vi "solar_type Message to Script.vi"(6 "Array Delimiters (1D,2D)":string[](array[string]), 7 "Type (CMD)":enum8{"CMD", "TLM"}(ring), 8 "error in (no error)":errorcluster, 9 "Data":variant, 10 "Packet":string, 11 "Target (\"\")":string) -> (0 "error out":errorcluster, 3 "String":string)   [LabVIEW 2018]
doc: "This converts a SOLAR variant message to script string. Formatted as:\n<b>CMD|TLM.TARGET:PACKET{\nTYPE:VALUE,\nTYPE:'VALUE',\nTYPE|ENUM0|ENUM1|...:VALUE,\nTYPE_1D:'1,2,3',\nTYPE_2D:'1,2,3;4,5,6'}</b>\n\n<b>TYPE</b>= I8, I16, I32, I64, U8, U16, U32, U64, U8_ENUM, U16_ENUM, U32_ENUM, SGL, DBL, BOOL, STR, PATH, TIME\nTYPE_1D: 1D array (comma ',' delimited) Ex: DBL_1D:'1.23,4.567,8.92'\nTYPE_2D: 2D array (comma ',' & semicolon ';' delimited) Ex: I32_2D:'1,2,3;4,5,6'\nTYPE_ENUM: Enum with type items (pipe '|' delimited) Ex: U16_ENUM|Item 1|Item 2|Item 3:'Item 2'\n\nMyTarget:MyCMD{\nI32:-1234,\nSTR:'Hello World',\nU16_ENUM|Item1|Item2|Item3:'Item2',\nBOOL:true,\nTIME:'yyyy-mm-dd_hh:mm:ss.uuuuuu',\nPATH:'C:\\Data\\test.txt',\nU8_2D:'1,2,3;4,5,6'}"
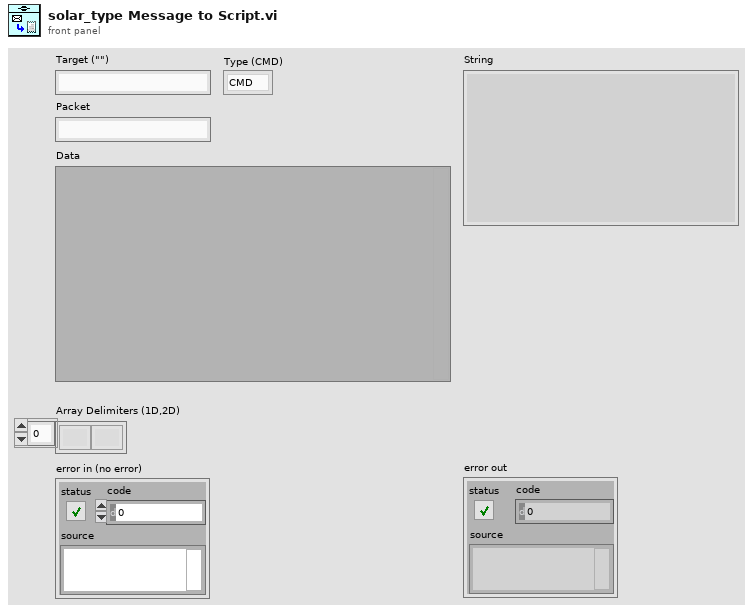
[diagram p1: front panel]
types:
  T1 = typedef "solar_type Item.ctl" = cluster{"Item":string, "Type":T2, "Value":variant, "States":string[]}
  T2 = typedef "solar_type Item Type.ctl" = enum16{"NULL", "UNKNOWN", "CLUSTER", "I8", "I16", "I32", "I64", "U8", "U16", "U32", "U64", "U8_ENUM", "U16_ENUM", "U32_ENUM", "SGL", "DBL", "BOOLEAN", "STRING", "PATH", "VISA", "TAG", "TIME", "I8_1D", "I16_1D", "I32_1D", "I64_1D", "U8_1D", "U16_1D", "U32_1D", "U64_1D", "U8_ENUM_1D", "U16_ENUM_1D", "U32_ENUM_1D", "SGL_1D", "DBL_1D", "BOOLEAN_1D", "STRING_1D", "PATH_1D", "VISA_1D", "TAG_1D", "TIME_1D", "I8_2D", "I16_2D", "I32_2D", "I64_2D", "U8_2D", "U16_2D", "U32_2D", "U64_2D", "U8_ENUM_2D", "U16_ENUM_2D", "U32_ENUM_2D", "SGL_2D", "DBL_2D", "BOOLEAN_2D", "STRING_2D", "PATH_2D", "VISA_2D", "TAG_2D", "TIME_2D"}
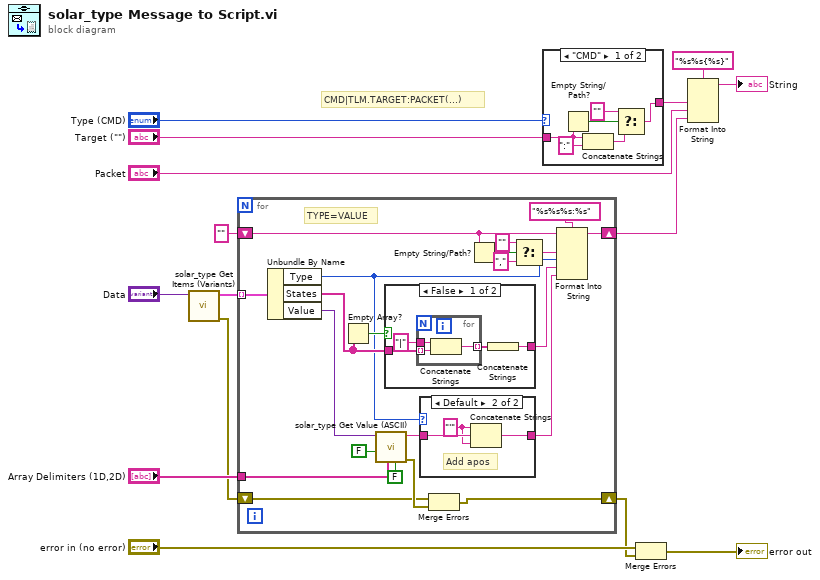
[diagram p0: block diagram]
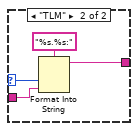
[diagram p2: hidden frame]
diagram:
  # "CMD|TLM.TARGET:PACKET(...)"
  n1 = call "solar_type Get Items (Variants).vi"("Variant"="Data") -> ("error out"=w2:errorcluster, "Items"=w6:T1[])  [unwired: 7 in, 2 out]
  n2 = for {
    tunnel: w6 -> [w36] mode=indexing
    tunnel: "Array Delimiters (1D,2D)" -> [w34]
    shift-right: [w29] -> w3
    shift-left: "" -> [w26]
    shift-right: [w17] -> w1
    shift-left: w2 -> [w16]
    # "TYPE=VALUE"
    n3 = Unbundle By Name(w36) -> ("Type"=w19:T2, "States"=w31:string[], "Value"=w33:variant)
    n4 = Empty Array?(array=w31) -> (empty?=w30:bool)
    n5 = call "solar_type Get Value (ASCII).vi"("Boolean as 0,1? (F)"=FALSE, "ArrayDelimiters (1D,2D)"=w34, "Use Enum Names? (F)"=FALSE, "Variant"=w33) -> ("error out"=w18:errorcluster, "Value (ASCII)"=w22:string)  [unwired: 5 in, 1 out]
    n6 = case shown="False" w30 {
      tunnel: w31 -> [w42 _]
      tunnel: [w41 _] -> w32
      frame False {
        n7 = for {
          tunnel: "|" ("delimiter (Tab)") -> [w47]
          tunnel: [w46] -> w43 mode=indexing
          tunnel: w42 -> [w45] mode=indexing
          n8 = Concatenate Strings(w47, w45) -> (w46:string)
        }
        n9 = Concatenate Strings(w43) -> (w41:string)
      }
      frame True {
      }
    }
    n10 = case shown="Default" w19 {
      tunnel: w22 -> [w37 w40]
      tunnel: [w37 w39] -> w21
      frame "I8".."U64", "SGL".."BOOLEAN" {
      }
      frame Default {
        w38 = "'" ("string")
        # "Add apos"
        n11 = Concatenate Strings(w38, w40, w38) -> (w39:string)
      }
    }
    n12 = Merge Errors(w16, w18) -> (w17:errorcluster)
    n13 = Empty String/Path?(string/path=w26) -> (empty?=w28:bool)
    n14 = Select(t="", s=w28, f=",") -> (s? t:f=w25:string)
    n15 = Format Into String(format string="%s%s%s:%s", initial string=w26, w25, w19, w32, w21) -> (resulting string=w29:string)  [unwired: 1 in, 1 out]
  }
  n16 = case shown="\"CMD\"" "Type (CMD)" {
    selector: "Type (CMD)" -> [_ w57]
    tunnel: "Target (\"\")" -> [w52 w55]
    tunnel: [w48 w54] -> w10
    frame "CMD" {
      n17 = Empty String/Path?(string/path=w52) -> (empty?=w53:bool)
      n18 = Concatenate Strings(w52, ":" ("string")) -> (w51:string)
      n19 = Select(t="", s=w53, f=w51) -> (s? t:f=w48:string)
    }
    frame "TLM" {
      n20 = Format Into String(format string="%s.%s:", w57, w55) -> (resulting string=w54:string)  [unwired: 2 in, 1 out]
    }
  }
  n21 = Merge Errors("error in (no error)", w1) -> (→"error out":errorcluster)
  n22 = Format Into String(format string="%s%s{%s}", w10, "Packet", w3) -> (resulting string=→"String":string)  [unwired: 2 in, 1 out]
